vi "state-ex1.vi"() -> ()   [LabVIEW 2013]
uses:
  Control 1.ctl
panel:
  in  "stop":bool
  out "motor on timer":u32
  out "milisecond timer":u32
  out "motor on":bool
  in  "motor timer [ms]":u32
  in  "user button":bool
  in  "index pulse":bool
  out "state":T1
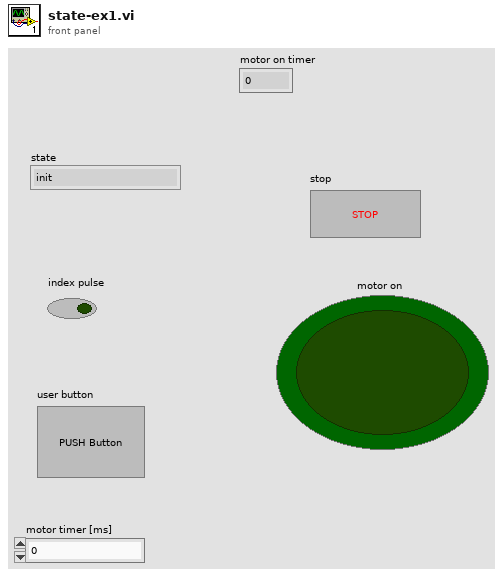
[diagram p1: front panel]
types:
  T1 = typedef "Control 1.ctl" = enum16{"init", "waiting for pulse", "waiting for button", "running motor", "shut down"}
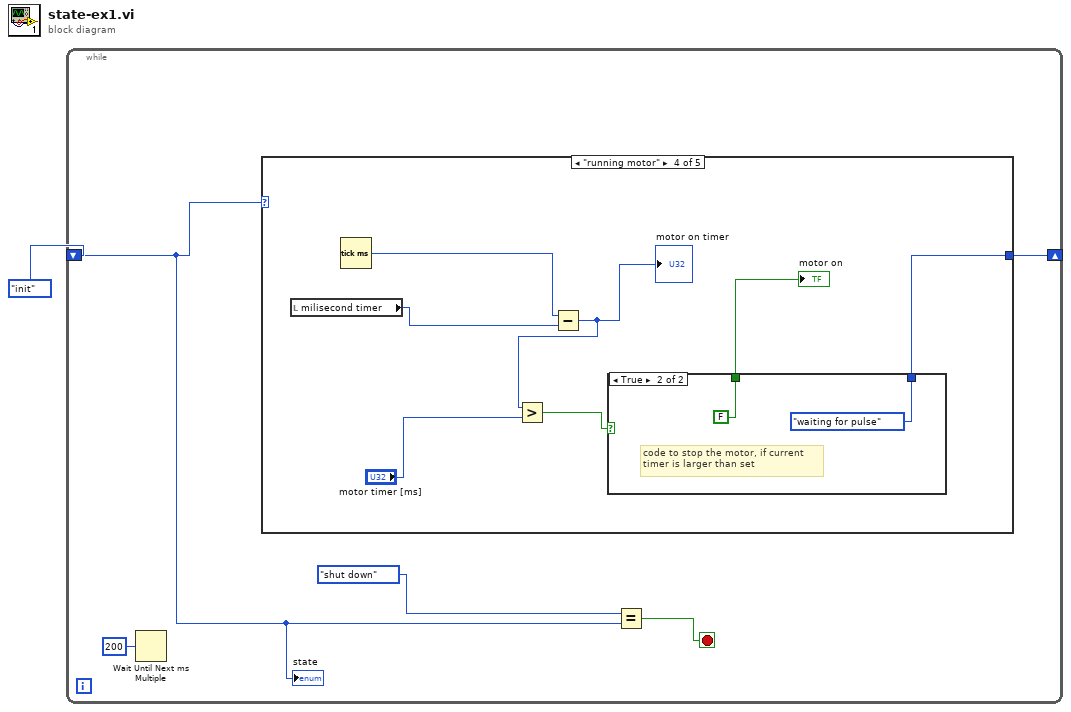
[diagram p0: block diagram]
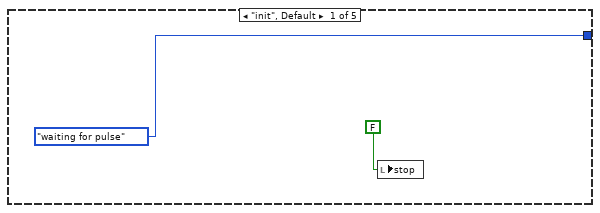
[diagram p2: hidden frame]
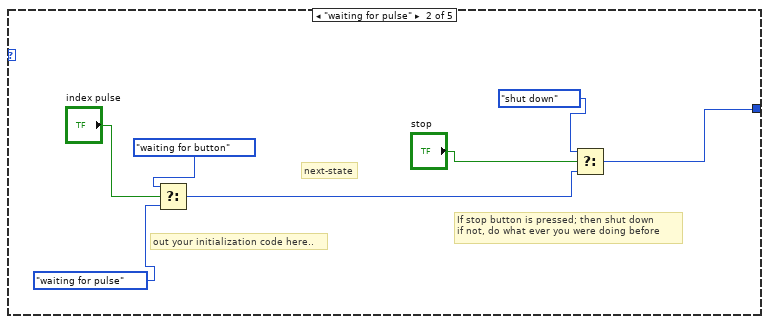
[diagram p3: hidden frame]
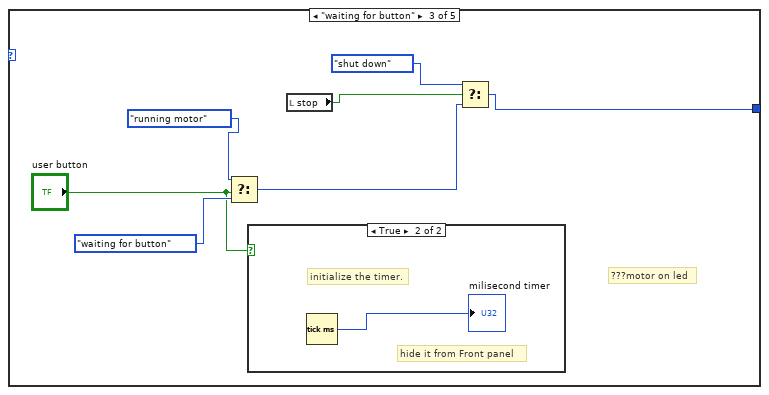
[diagram p4: hidden frame]
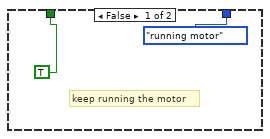
[diagram p6: hidden frame]
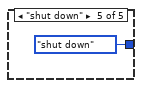
[diagram p7: hidden frame]
diagram:
  n1 = while {
    shift-right: [w3] -> _
    shift-left: Control_1."init" ("state") -> [w4]
    stop <- w5 stop-if-true
    n2 = Wait Until Next ms Multiple(millisecond multiple=u32 200) -> ()  [unwired: 1 out]
    n3 = case shown="\"running motor\"" w4 {
      tunnel: [Control_1."waiting for pulse" ("state") w9 w17 w27 Control_1."shut down" ("state")] -> w3
      frame "init", Default {
        n4 = local write "stop"(FALSE ("stop")) -> ()
      }
      frame "waiting for pulse" {
        # "If stop button is pressed; then shut down\nif not, do what ever you were doing before"
        # "out your initialization code here.."
        # "next-state"
        n5 = Select(t=Control_1."waiting for button" ("state"), s="index pulse", f=Control_1."waiting for pulse" ("state")) -> (s? t:f=w11:T1)
        n6 = Select(t=Control_1."shut down" ("state"), s="stop", f=w11) -> (s? t:f=w9:T1)
      }
      frame "waiting for button" {
        # "???motor on led"
        n7 = Select(t=Control_1."running motor" ("state"), s="user button", f=Control_1."waiting for button" ("state")) -> (s? t:f=w19:T1)
        n8 = case shown="True" "user button" {
          frame False {
          }
          frame True {
            # "hide it from Front panel"
            # "initialize the timer."
            n9 = Tick Count (ms)() -> (millisecond timer value=→"milisecond timer":u32)
          }
        }
        n10 = local read "stop"() -> (w16:bool)
        n11 = Select(t=Control_1."shut down" ("state"), s=w16, f=w19) -> (s? t:f=w17:T1)
      }
      frame "running motor" {
        n12 = local read "milisecond timer"() -> (w24:u32)
        n13 = Tick Count (ms)() -> (millisecond timer value=w25:u32)
        n14 = Subtract(x=w25, y=w24) -> (x-y=w30:u32)
        "motor on timer" <- w30
        n15 = Greater?(x=w30, y="motor timer [ms]") -> (0:w28:bool)
        n16 = case shown="True" w28 {
          tunnel: [TRUE FALSE] -> w26
          tunnel: [Control_1."running motor" ("state") Control_1."waiting for pulse" ("state")] -> w27
          frame False {
            # "keep running the motor"
          }
          frame True {
            # "code to stop the motor, if current \ntimer is larger than set"
          }
        }
        "motor on" <- w26
      }
      frame "shut down" {
      }
    }
    n17 = Equal?(x=Control_1."shut down" ("state"), y=w4) -> (x = y?=w5:bool)
    "state" <- w4
  }
